vi "Find Contact.vi"(8 "error in (no error)":errorcluster, 10 "ID":u32, 11 "All Lines":T1) -> (0 "error out":errorcluster, 2 "Index":i32, 3 "All Lines 2":T1)   [LabVIEW 2014, in "Map Data.lvlib"]
doc: "Searches the data store for a single contact by ID."
uses:
  Map Data.lvlib
  All-Lines.ctl
  LineCluster.ctl
  LineConnection.ctl
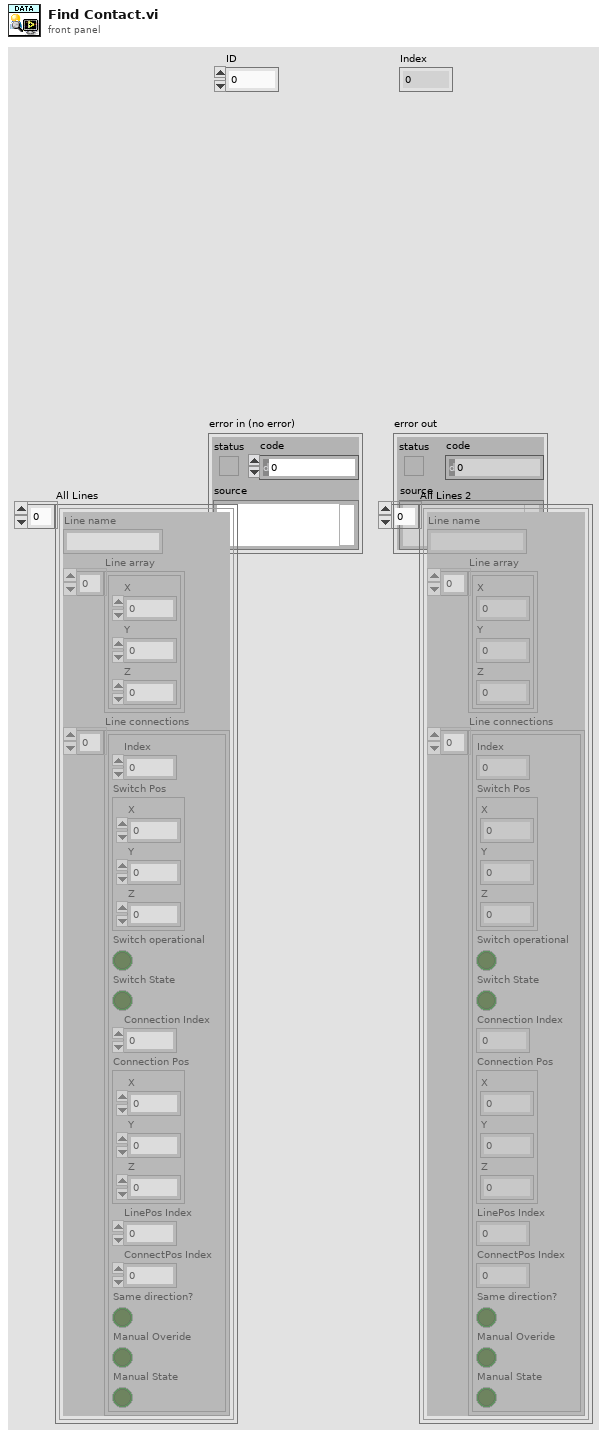
[diagram p1: front panel]
types:
  T1 = typedef "Map Data.lvlib/All-Lines.ctl" = T2[]
  T2 = typedef "Map Data.lvlib/LineCluster.ctl" = cluster{"Line name":string, "Line array":cluster{"X":dbl, "Y":dbl, "Z":dbl}[], "Line connections":T3[]}
  T3 = typedef "LineConnection.ctl" = cluster{"Index":i32, "Switch Pos":cluster{"X":dbl, "Y":dbl, "Z":dbl}, "Switch operational":bool, "Switch State":bool, "Connection Index":i32, "Connection Pos":cluster{"X":dbl, "Y":dbl, "Z":dbl}, "LinePos Index":i32, "ConnectPos Index":i32, "Same direction?":bool, "Manual Overide":bool, "Manual State":bool}
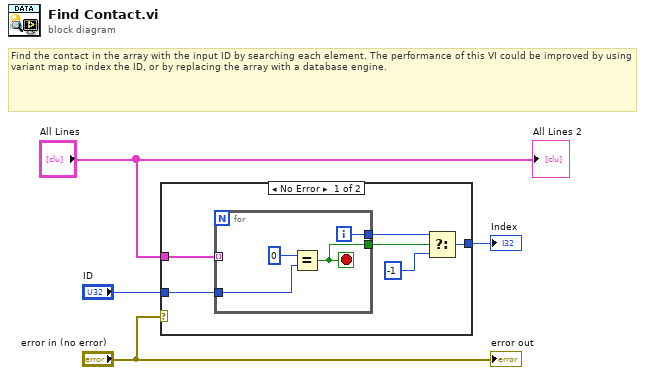
[diagram p0: block diagram]
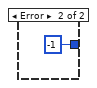
[diagram p2: hidden frame]
diagram:
  # "Find the contact in the array with the input ID by searching each element. The performance of this VI could be improved by using variant map to index the ID, or by replacing the array with a database engine."
  n1 = case shown="No Error" "error in (no error)" {
    tunnel: "ID" -> [w10 _]
    tunnel: "All Lines" -> [w9 _]
    tunnel: [w5 -1 ("f")] -> w3
    frame No Error {
      n2 = for {
        tunnel: w9 -> [_] mode=indexing
        tunnel: w10 -> [w14]
        tunnel: [w13] -> w7
        tunnel: [w12] -> w8
        i -> [w13]
        stop <- w12 stop-if-true
        n3 = Equal?(x=u32 0, y=w14) -> (x = y?=w12:bool)
      }
      n4 = Select(t=w7, s=w8, f=-1) -> (s? t:f=w5:i32)
    }
    frame Error {
    }
  }
  "Index" <- w3
  "error out" <- "error in (no error)"
  "All Lines 2" <- "All Lines"
